vi "leerTupla.vi"(6 "error in":errorcluster, 11 "tableName":string) -> (0 "error out":errorcluster, 2 "arrayNamesFullOut":string[](array[string]), 3 "dataReadingOut":string[][](array[string]))   [LabVIEW 2014]
uses:
  <vilib>/addons/database/Connection.llb/DB Tools Open Connec (String).vi
  <vilib>/addons/database/NI_Database_API.lvlib
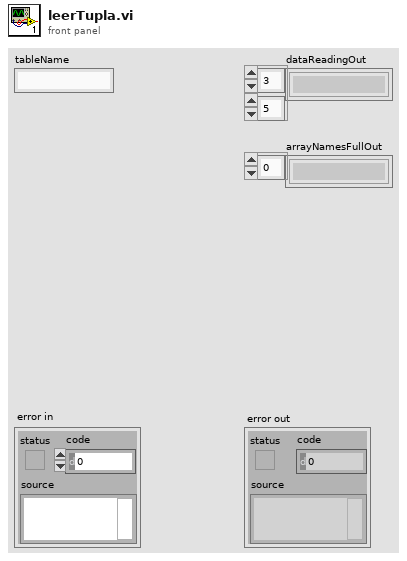
[diagram p1: front panel]
types:
  T1 = typedef "NI_Database_API.lvlib/Conn ObjectReference.ctl" = refnum<k1>
  T2 = typedef "NI_Database_API.lvlib/DB Tools DataTypes.ctl" = enum16{"String", "Long (I32)", "Single (SGL)", "Double (DBL)", "Date/Time", "Binary"}
  T3 = cluster{"name":string, "database data type":T2, "defined size":i32}[]
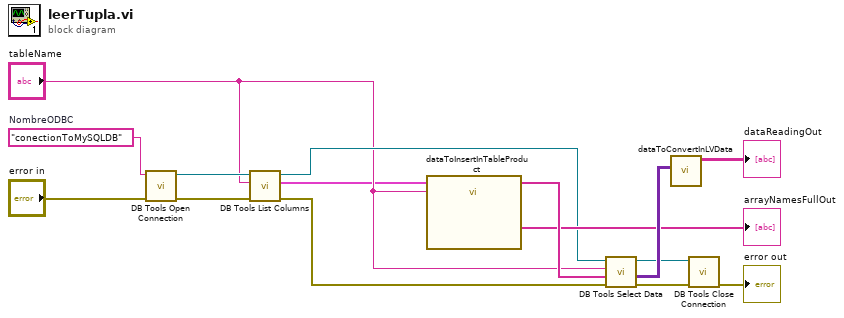
[diagram p0: block diagram]
diagram:
  w11 = "conectionToMySQLDB"  # NombreODBC
  n1 = call-poly <vilib>:"DB Tools Open Connection.vi"("error in (no error)"="error in", "connection information"=w11) -> ("error out"=w9:errorcluster, "connection reference"=w10:T1)  [unwired: 6 in]
  n2 = call <vilib>:"DB Tools List Columns.vi"("error in (no error)"=w9, "table"="tableName", "connection reference"=w10) -> ("error out"=w7:errorcluster, "column information"=w1:T3, "connection reference out"=w6:T1)  [unwired: 1 in, 1 out]
  n3 = call "dataToInsertInTableProduct.vi"("arrayNamesInTableIN"=w1, "tableIn"="tableName") -> ("arrayNamesInTableOUT"=w15:string[], "arrayNamesFullOut"=→"arrayNamesFullOut":string[])  [unwired: 7 in, 5 out]
  n4 = call <vilib>:"DB Tools Select Data.vi"("error in (no error)"=w7, "columns"=w15, "table"="tableName", "connection reference"=w6) -> ("error out"=w5:errorcluster, "data"=w14:variant[][], "connection reference out"=w3:T1)  [unwired: 2 in]
  n5 = call "dataToConvertInLVData.vi"("dataReadingIn"=w14) -> ("dataReadingOut"=→"dataReadingOut":string[][])  [unwired: 9 in, 1 out]
  n6 = call <vilib>:"DB Tools Close Connection.vi"("error in (no error)"=w5, "connection reference"=w3) -> ("error out"=→"error out":errorcluster)  [unwired: 5 in]
